vi "GETPORTSTATUS.vi"(8 "error in (no error)":errorcluster, 10 "Port to read":dbl, 11 "NXP in":refnum<class "NXP.lvclass">) -> (0 "error out":errorcluster, 3 "NXP out":refnum<class "NXP.lvclass">)   [LabVIEW 2019, in "NXP.lvclass"]
uses:
  NXP.lvclass
  NXP.lvclass/NXP.ctl
  d1acd0f8-f0fb-4928-889e-17536973e7db.vi
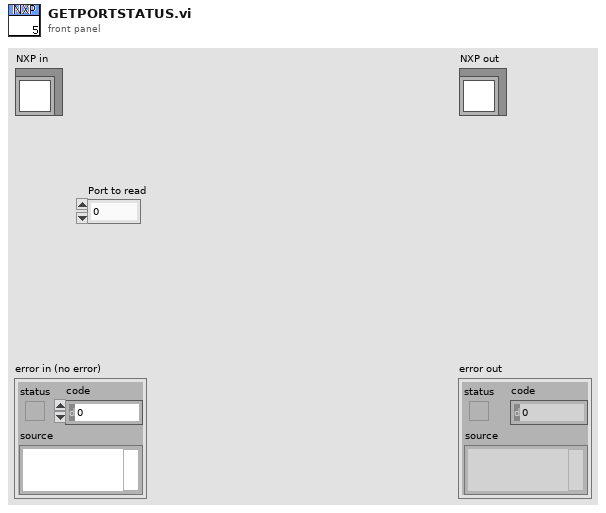
[diagram p1: front panel]
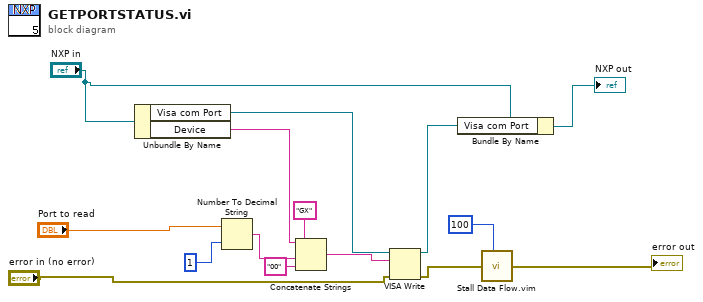
[diagram p0: block diagram]
diagram:
  n1 = Unbundle By Name("NXP in") -> ("Visa com Port"=w13:refnum<visa-resource-name>, "Device"=w12:string)
  n2 = Number To Decimal String(number="Port to read", width (-)=i16 1) -> (decimal integer string=w10:string)
  n3 = Concatenate Strings(w12, "GX" ("string"), w10, "00" ("string")) -> (w8:string)
  n4 = VISA Write(VISA resource name=w13, write buffer=w8, error in (no error)="error in (no error)") -> (VISA resource name out=w1:refnum<visa-resource-name>, error out=w6:errorcluster)  [unwired: 1 out]
  n5 = Bundle By Name(cluster="NXP in", "Visa com Port"=w1) -> (→"NXP out":refnum<class "NXP.lvclass">)
  n6 = call "Stall Data Flow.vim"("value in"=w6, "milliseconds to wait"=u32 100) -> ("value out"=→"error out":errorcluster)  [unwired: 1 out]
